vi "imp_test_v3.vi"() -> ()   [LabVIEW 2014]
uses:
  <vilib>/LabVIEW Targets/FPGA/cRIO/shared/nicrio_ModuleControls/nicrio_cRIO-9237_DataRatesRing.ctl
  <vilib>/LabVIEW Targets/FPGA/cRIO/shared/nicrio_ModuleControls/nicrio_cRIO-9237_ExcitationVoltageRing.ctl
  <vilib>/rvi/FXPMathLib/FxpSinAndCos/subVIs/nifxpmath_SinAndCos_SimConfig.ctl
  <vilib>/rvi/Emulation/niFpgaGetClockAttributes.vi
  <vilib>/rvi/Emulation/niFpgaSctlEmulationGetInTimedLoop.vi
  <vilib>/rvi/Emulation/niFpgaEmulationReportErrorSimple.vi
  <vilib>/rvi/Emulation/niFpgaProcessEmulError.vi
  <vilib>/rvi/interface/RandomDataEmulation/nirviRandomDataMultiElementFPGAFIFO.vi
  <instcachedir>/0/nirviRandomDataMultiElementFPGAFIFO_AD0CFC12EF974623A9C2E4184BC062B2.lvgen/nirviRandomDataMultiElementFPGAFIFO_AD0CFC12EF974623A9C2E4184BC062B2_023.vi
  <vilib>/rvi/interface/RandomDataEmulation/niFpgaRandomDataHandleErrors.vi
  <vilib>/rvi/Emulation/niFpgaCriticalErrorInLSC.vi
  <vilib>/rvi/eio/common/nirviEmuTemplateMethod_errors.vi
  <vilib>/rvi/FXPMathLib/FxpSinAndCos/simVIs/DllFxpSinAndCosTemp_sub.vi
  <vilib>/rvi/eio/common/nirviEmuTemplatePropertySet_errors.vi
  <vilib>/rvi/DataTransferAndStorage/Container/XNode/niFpgaContainer.xnode
  <vilib>/rvi/interface/RandomDataEmulation/nirviRandomDataFpgaMultiElementTemplate.vi
  <vilib>/eio/EIONode/EIONode.xnode
  <vilib>/rvi/FXPMathLib/FxpMul/XNode/nifxpmath_Multiplier.xnode
  <vilib>/rvi/FXPMathLib/FxpSinAndCos/XNode/nifxpmath_SinAndCos.xnode
  <vilib>/rvi/Analysis/measure/butterworth/XNode/niFpgaButterworthFilter.xnode
  <vilib>/rvi/FXPMathLib/FxpSub/XNode/nifxpmath_Sub.xnode
  <vilib>/rvi/FXPMathLib/FxpAdd/XNode/nifxpmath_Add.xnode
  <vilib>/eio/EIOPropertyNode/EIOPropertyNode.xnode
  <vilib>/rvi/eio/common/nirviEmuTemplatePropertyGet_errors.vi
  <vilib>/rvi/eio/common/nirviEmuTemplatePropertyGet_noerrors.vi
  <vilib>/rvi/eio/common/nirviEmuTemplatePropertySet_noerrors.vi
  <vilib>/rvi/FXPMathLib/sim/FxpSim.dll
panel:
  out "Strain (mf)":fxp<+/-,36,8>
  in  "Strain mean coeff.":i32[](array[numeric])=[-898916953, 1957103773, 3888751]
  out "Dr_for":fxp<+/-,39,10>
  in  "Command type":i16(ring) items=["Step", "Sine"]
  out "Strain (mean)":fxp<+/-,32,4>
  in  "Strain selection":i16(ring) items=["Raw strain", "Mean strain", "Mean strain (f)", "Filtered strain"]
  in  "ft_d or dt_d2":i16(ring) items=["ft_d", "ft_d2"]
  out "vb":fxp<+/-,38,8>
  out "va":fxp<+/-,38,8>
  out "ft_d2":fxp<+/-,64,59>
  out "Force_r":fxp<+/-,64,42>
  in  "Bv":fxp<+/-,22,8>
  out "D_error_dd":fxp<+/-,64,49>
  out "D_error_d":fxp<+/-,33,10>
  in  "Kv":fxp<+/-,22,8>
  out "D_error":fxp<+/-,64,33>
  out "Dr_sin_dd":fxp<+/-,64,48>
  out "Dr_sin_d":fxp<+/-,64,17>
  out "Sin omega":fxp<+/-,52,9>
  out "Dr_sin":fxp<+/-,39,10>
  in  "Sin offset":fxp<+/-,38,9>
  in  "Sin magnitude":fxp<+/-,22,7>
  out "Time now(s)":fxp<+,52,14>
  in  "Sin wave freq. (Hz)":fxp<+/-,32,6>
  in  "Dr_step":fxp<+/-,22,7>
  in  "Drive mode":i16(ring) items=["Backward", "Forward"]
  in  "ft_d coeff.":i32[](array[numeric])=[946630756, 63555534]
  out "ft_d":fxp<+/-,36,25>
  out "D_dd":fxp<+/-,36,24>
  in  "D_dd coeff.":i32[](array[numeric])=[946630756, 63555534]
  out "dF_PID":fxp<+/-,36,33>
  in  "dF_PID coeff.":i32[](array[numeric])=[946630756, 63555534]
  out "ft_i":fxp<+/-,34,18>
  out "F_PID":fxp<+/-,51,14>
  in  "f_tolorance":fxp<+,22,6>
  in  "Ki":fxp<+/-,36,9>
  in  "Kd":fxp<+/-,36,9>
  out "f_tilde":fxp<+/-,33,11>
  in  "Kp":fxp<+/-,36,9>
  out "vq_F":fxp<+/-,20,5> format="%.57g"
  out "vd_F":fxp<+/-,20,5>
  in  "dF_add":bool
  out "D_d(mm/s)":fxp<+/-,41,10>
  out "omega(rad/s)":fxp<+/-,20,9>
  in  "Veolcity Estimation":i16(ring) items=["T method", "M_avg method", "M method"]
  in  "Stop motor":bool
  out "D_d(T)":fxp<+/-,41,10>
  out "omega(T)":fxp<+/-,20,9>
  in  "mt0_omega":u32
  out "mt_omega":u32
  out "rad(NrTheta)":fxp<+/-,33,20>
  out "D(mm)":fxp<+/-,32,10>
  out "Encoder Position":i32
  in  "Encoder reset":bool
  in  "Ini coe.":bool
  out "Loop rate (kHz)":fxp<+/-,36,7>
  in  "Strain filter coeff.":i32[](array[numeric])=[-850883994, 1909449570, 3794062, -975456236, 2033039520, 4039635]
  out "Force":fxp<+/-,32,10>
  out "Strain (filter)":fxp<+/-,36,4>
  out "Fileterd data":fxp<+/-,32,4>
  in  "S/F coeff":fxp<+/-,20,-12>
  out "Raw Strain":fxp<+/-,36,4>
  in  "Strain gage reset":bool
  in  "Stop (Strain)":bool
  out "Mod6/AI2":fxp<+/-,32,4>
  in  "Shunt Cal Enable":bool
  in  "Half-Bridge Enable":bool
  in  "Excitation Voltage":T1 items=["2.5 Volts", "3.3 Volts", "5.0 Volts", "10.0 Volts", "External Excitation"]
  in  "Data Rate":T2=1 items=["50.000 kS/s (NI 9237)"=1, "25.000 kS/s (NI 9237)"=2, "16.667 kS/s (NI 9237)"=3, "12.500 kS/s (NI 9237)"=4, "10.000 kS/s (NI 9237)"=5, "8.333 kS/s (NI 9237)"=6, "7.143 kS/s (NI 9237)"=7, "6.250 kS/s (NI 9237)"=8, "5.556 kS/s (NI 9237)"=9, "5.000 kS/s (NI 9237)"=10, "4.545 kS/s (NI 9237)"=11, "4.167 kS/s (NI 9237)"=12, "3.846 kS/s (NI 9237)"=13, "3.571 kS/s (NI 9237)"=14, "3.333 kS/s (NI 9237)"=15, "3.125 kS/s (NI 9237)"=16, "2.941 kS/s (NI 9237)"=17, "2.778 kS/s (NI 9237)"=18, "2.632 kS/s (NI 9237)"=19, "2.500 kS/s (NI 9237)"=20, "2.381 kS/s (NI 9237)"=21, "2.273 kS/s (NI 9237)"=22, "2.174 kS/s (NI 9237)"=23, "2.083 kS/s (NI 9237)"=24, "2.000 kS/s (NI 9237)"=25, "1.923 kS/s (NI 9237)"=26, "1.852 kS/s (NI 9237)"=27, "1.786 kS/s (NI 9237)"=28, "1.724 kS/s (NI 9237)"=29, "1.667 kS/s (NI 9237)"=30, "1.613 kS/s (NI 9237)"=31]
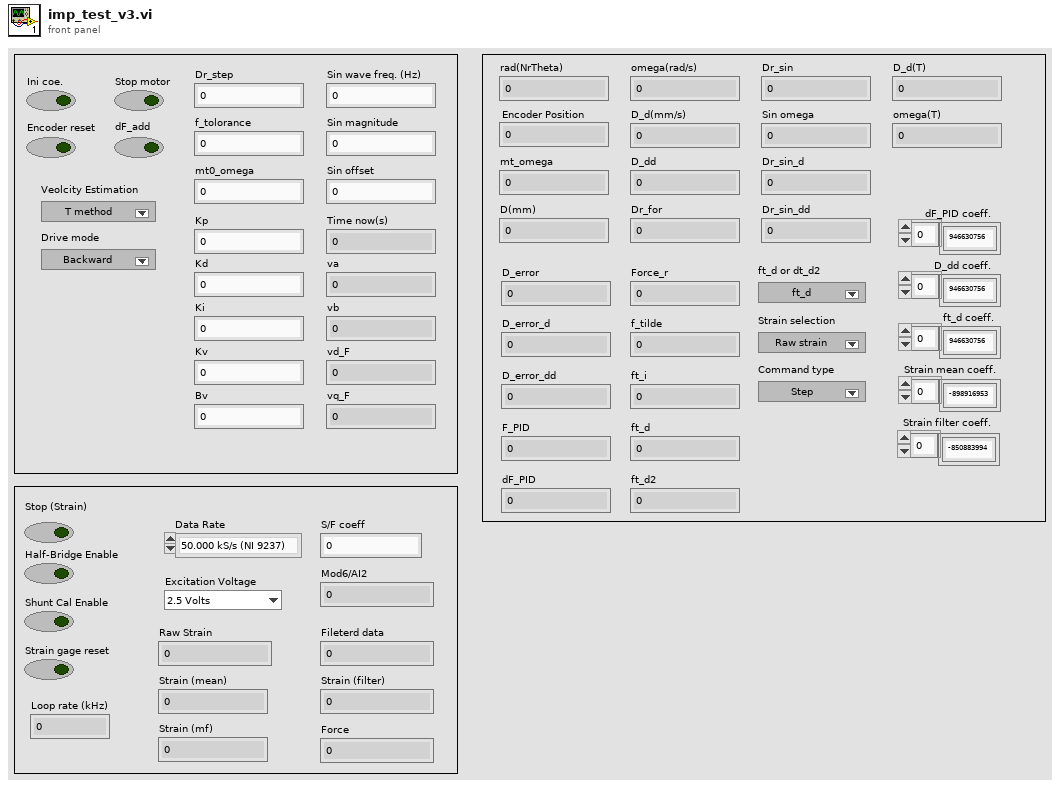
[diagram p1: front panel]
types:
  T1 = typedef "nicrio_cRIO-9237_ExcitationVoltageRing.ctl" = u8
  T2 = typedef "nicrio_cRIO-9237_DataRatesRing.ctl" = u8
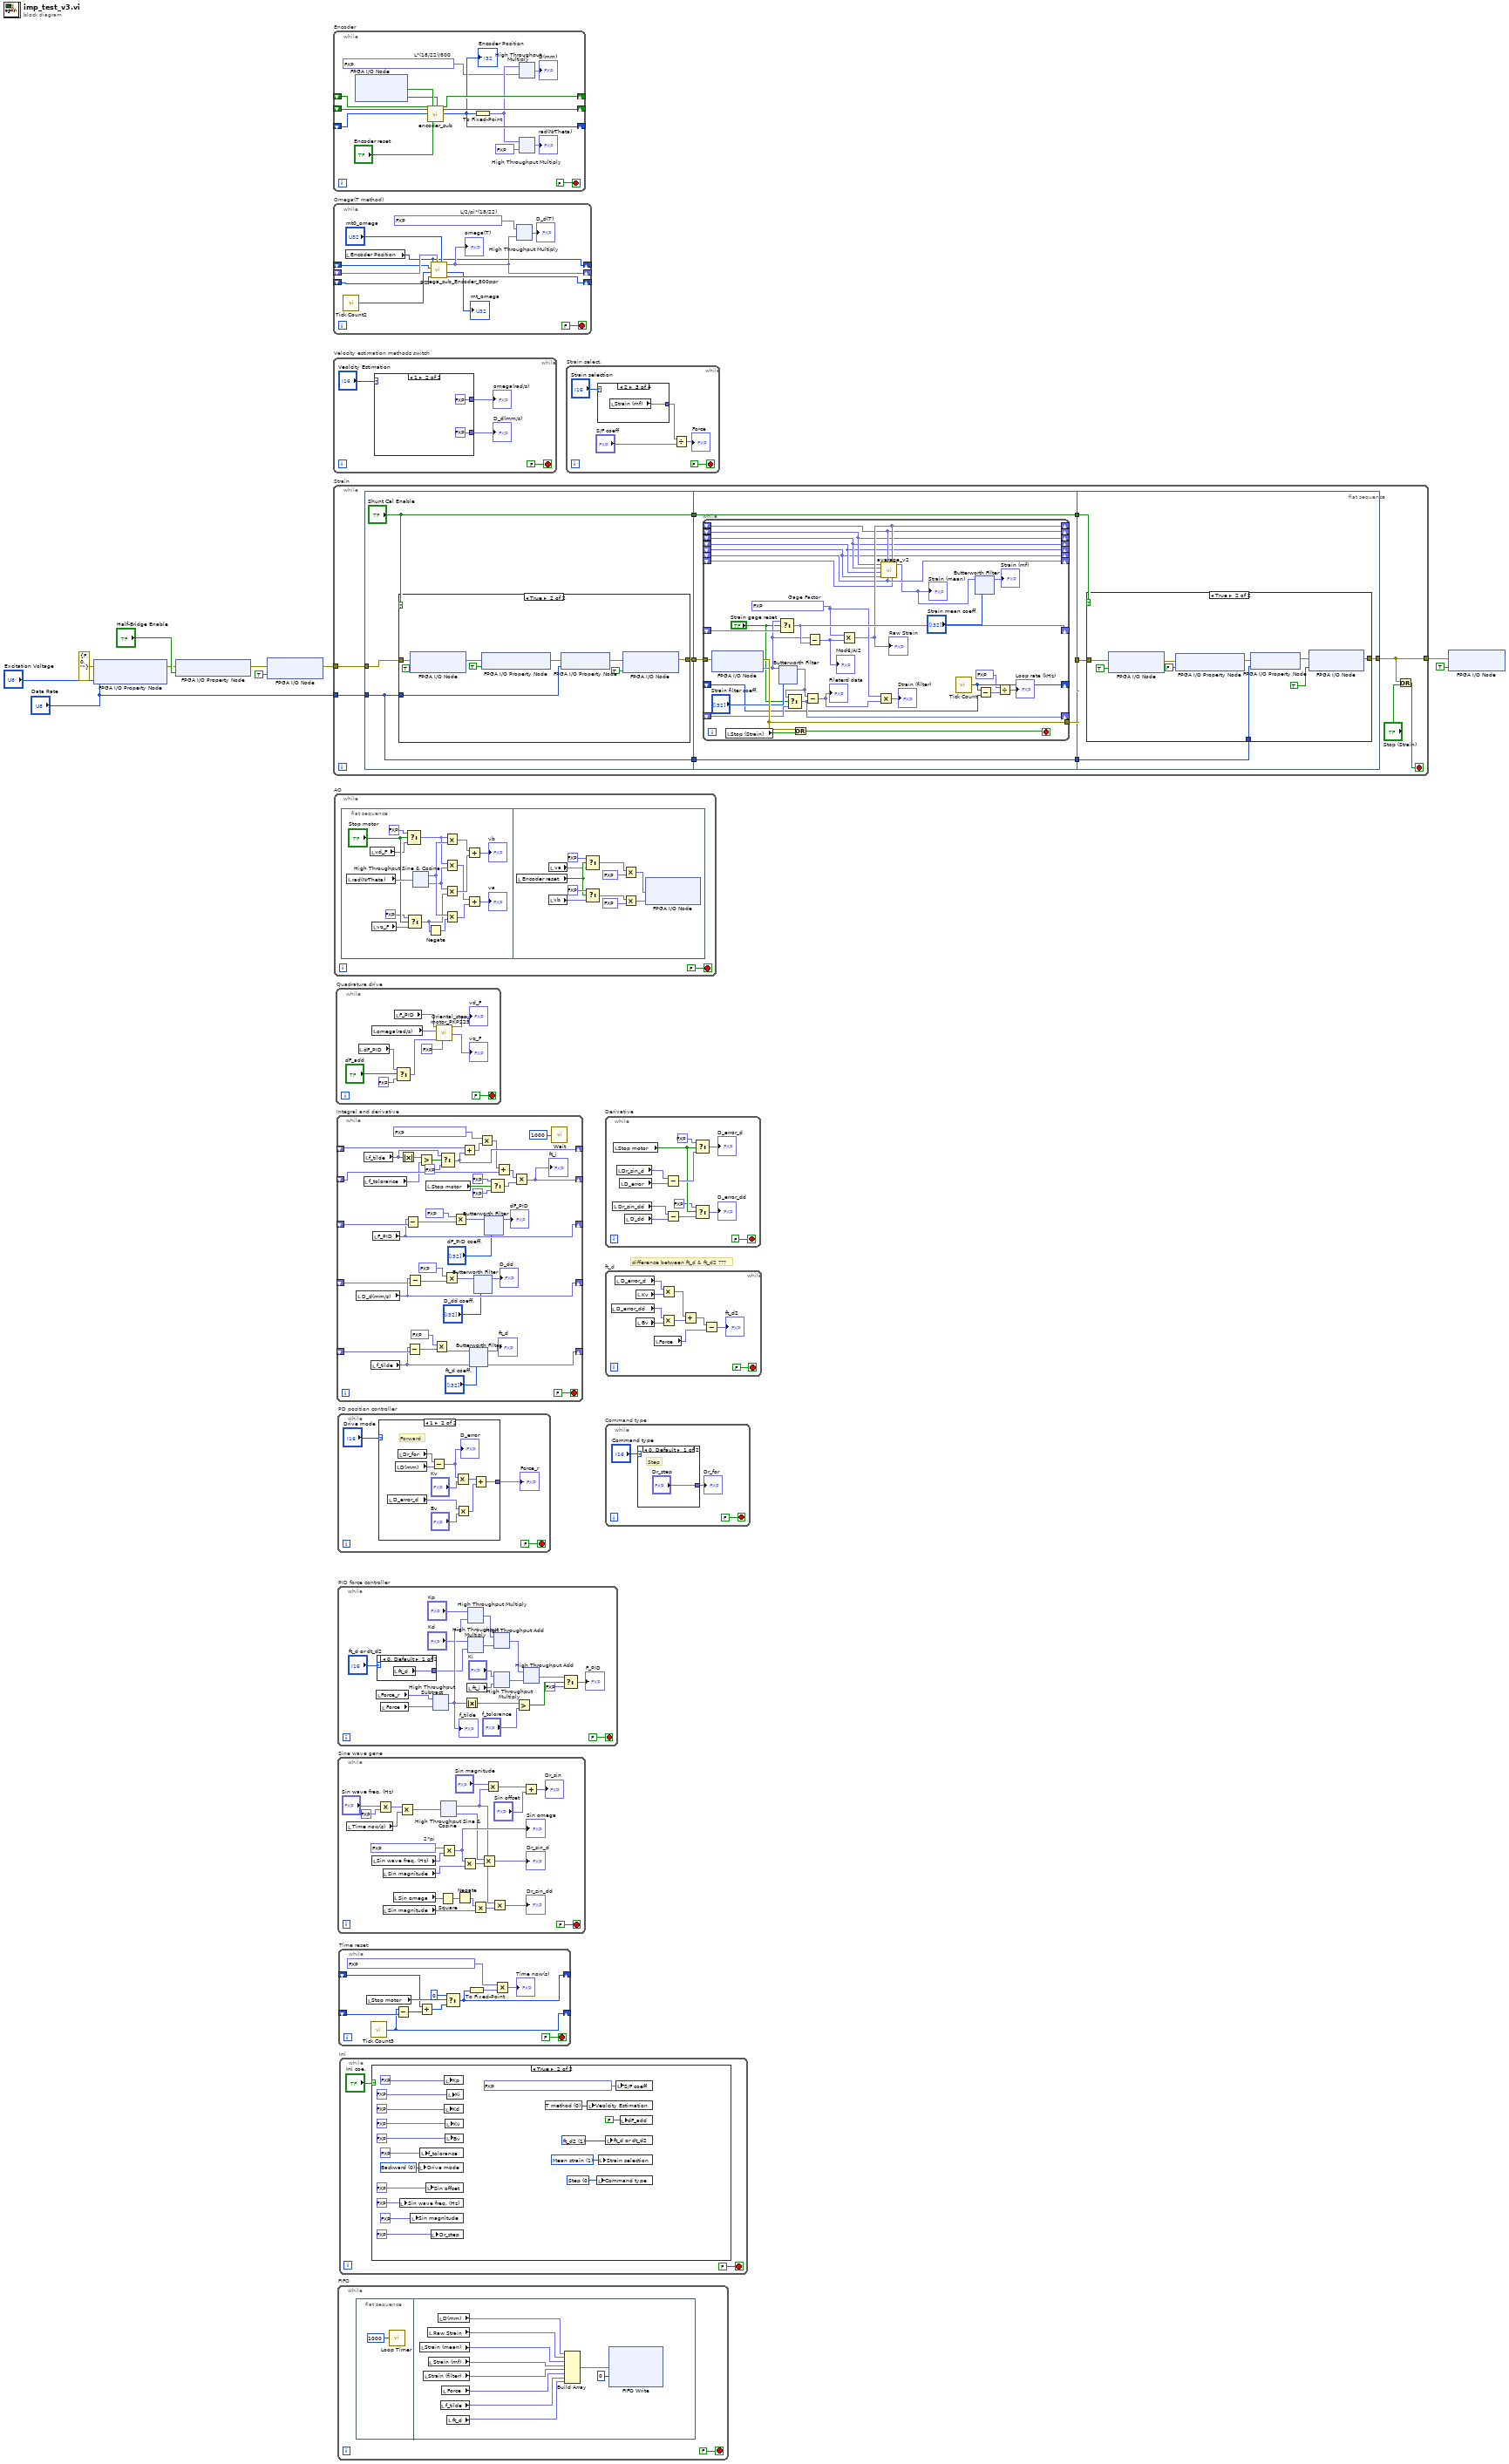
[diagram p0: block diagram]
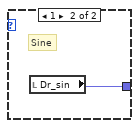
[diagram p2: hidden frame]
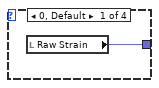
[diagram p3: hidden frame]
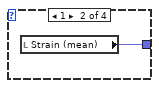
[diagram p4: hidden frame]
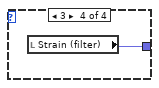
[diagram p5: hidden frame]
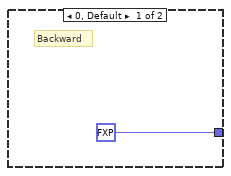
[diagram p6: hidden frame]
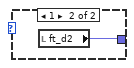
[diagram p7: hidden frame]
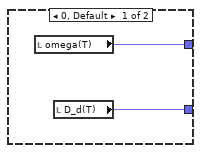
[diagram p8: hidden frame]
diagram:
  # "difference between ft_d & ft_d2 ???"
  n1 = xnode "FPGA I/O Property Node"("error in"=errorcluster {"status"=FALSE, "code"=0, "source"=""}, "Data Rate"="Data Rate", "Excitation Voltage"="Excitation Voltage") -> ("error out"=w7:errorcluster)  [unwired: 1 in, 1 out]
  n2 = xnode "FPGA I/O Property Node"("error in"=w7, "Half-Bridge Enable"="Half-Bridge Enable") -> ("error out"=w6:errorcluster)  [unwired: 1 in, 1 out]
  n3 = xnode "FPGA I/O Node"("error in"=w6, "Mod6/Start"=TRUE) -> ("error out"=w4:errorcluster)  [unwired: 1 in, 1 out]
  n4 = while "Encoder" {
    shift-right: [w22] -> _
    shift-left: _ -> [w23]
    shift-right: [w24] -> _
    shift-left: _ -> [w25]
    shift-right: [w17] -> _
    shift-left: _ -> [w21]
    stop <- FALSE stop-if-true
    w14 = fxp<+/-,32,0> 0.0020454544574022293  # L*(18/22)/800
    n5 = xnode "FPGA I/O Node"() -> ("Mod4/DI3"=w20:bool, "Mod4/DI4"=w19:bool)  [unwired: 2 in, 2 out]
    n6 = call "encoder_sub.vi"("A_pre"=w23, "B_pre"=w25, "Encoder Position_pre"=w21, "A input"=w20, "Encoder Position Reset"="Encoder reset", "B input"=w19) -> ("A"=w22:bool, "B"=w24:bool, "Encoder Position (Counts)"=w17:i32)  [unwired: 19 in]
    "Encoder Position" <- w17
    n7 = To Fixed-Point(number=w17) -> (fixed-point=w16:fxp<+/-,32,32>)  [unwired: 1 in]
    n8 = xnode ("High Throughput Multiply")("x"=w16, "y"=w14) -> ("x*y"=→"D(mm)":fxp<+/-,64,32>)
    n9 = xnode ("High Throughput Multiply")("x"=w16, "y"=fxp<+/-,16,1> 0.125) -> ("x*y"=→"rad(NrTheta)":fxp<+/-,48,33>)
  }
  n10 = while "Omega(T method)" {
    shift-right: [w27] -> _
    shift-left: _ -> [w28]
    shift-right: [w31] -> _
    shift-left: _ -> [w33]
    shift-right: [w35] -> _
    shift-left: _ -> [w36]
    stop <- FALSE stop-if-true
    w30 = fxp<+/-,32,0> 0.2604353614151478  # L/2/pi*(18/22)
    n11 = call "Tick Count2"() -> ("Tick Count(Ticks)"=w37:u32)
    n12 = local read "Encoder Position"() -> (w27:i32)
    n13 = call "omega_sub_Encoder_800ppr.vi"("mt0"="mt0_omega", "omega_pre"=w33, "ticks_m_pre"=w36, "ticks"=w37, "count_pre"=w28, "count"=w27) -> ("ticks_m"=w35:u32, "mt"=→"mt_omega":u32, "omega"=w31:fxp<+/-,20,9>)  [unwired: 3 in]
    "omega(T)" <- w31
    n14 = xnode ("High Throughput Multiply")("x"=w30, "y"=w31) -> ("x*y"=→"D_d(T)":fxp<+/-,52,9>)
  }
  n15 = while "Velocity estimation methods switch" {
    stop <- FALSE stop-if-true
    n16 = case shown="1" "Veolcity Estimation" {
      tunnel: [w43 fxp<+/-,20,9> 0.0 ("omega(T)")] -> w40
      tunnel: [w42 fxp<+/-,41,10> 0.0 ("D_d(T)")] -> w39
      frame 0, Default {
        n17 = local read "omega(T)"() -> (w43:fxp<+/-,20,9>)
        n18 = local read "D_d(T)"() -> (w42:fxp<+/-,41,10>)
      }
      frame 1 {
      }
    }
    "omega(rad/s)" <- w40
    "D_d(mm/s)" <- w39
  }
  n19 = while "Strain" {
    tunnel: w4 -> [w56]
    tunnel: "Data Rate" -> [w55]
    tunnel: [w47] -> w2
    stop <- w48 stop-if-true
    n20 = flat-sequence {
      tunnel: w56 -> [w60]
      tunnel: w55 -> [w59]
      tunnel: [w59] -> w54
      tunnel: ["Shunt Cal Enable"] -> w53
      tunnel: [w57] -> w52
      tunnel: w54 -> [w72]
      tunnel: w53 -> [w73]
      tunnel: w52 -> [w74]
      tunnel: [w73] -> w51
      tunnel: [w71] -> w50
      tunnel: [w72] -> w49
      tunnel: w51 -> [w126]
      tunnel: w50 -> [w125]
      tunnel: w49 -> [w124]
      tunnel: [w123] -> w47
      frame #0 {
        n21 = case shown="True" "Shunt Cal Enable" {
          tunnel: w60 -> [w61 w68]
          tunnel: w59 -> [_ w66]
          tunnel: [w61 w63] -> w57
          frame False {
          }
          frame True {
            n22 = xnode "FPGA I/O Node"("error in"=w68, "Mod6/Stop"=TRUE) -> ("error out"=w69:errorcluster)  [unwired: 1 in, 1 out]
            n23 = xnode "FPGA I/O Property Node"("error in"=w69, "Shunt Cal Enable"=TRUE) -> ("error out"=w67:errorcluster)  [unwired: 1 in, 1 out]
            n24 = xnode "FPGA I/O Property Node"("error in"=w67, "Data Rate"=w66) -> ("error out"=w65:errorcluster)  [unwired: 1 in, 1 out]
            n25 = xnode "FPGA I/O Node"("error in"=w65, "Mod6/Start"=TRUE) -> ("error out"=w63:errorcluster)  [unwired: 1 in, 1 out]
          }
        }
      }
      frame #1 {
        n26 = while {
          tunnel: w74 -> [w106]
          tunnel: [w104] -> w71
          shift-right: [w102] -> _
          shift-left: _ -> [w103]
          shift-right: [w98] -> _
          shift-left: _ -> [w99]
          shift-right: [w90] -> _
          shift-left: _ -> [w91]
          shift-right: [w85] -> _
          shift-left: _ -> [w84]
          shift-right: [w84] -> _
          shift-left: _ -> [w83]
          shift-right: [w83] -> _
          shift-left: _ -> [w82]
          shift-right: [w82] -> _
          shift-left: _ -> [w81]
          shift-right: [w81] -> _
          shift-left: _ -> [w80]
          shift-right: [w80] -> _
          shift-left: _ -> [w79]
          shift-right: [w79] -> _
          shift-left: _ -> [w78]
          stop <- w93 stop-if-true
          w96 = fxp<+,20,2> 2.115001678466797  # Gage Factor
          n27 = xnode "FPGA I/O Node"("error in"=w106) -> ("error out"=w104:errorcluster, "Mod6/AI2"=w100:fxp<+/-,24,-4>)  [unwired: 1 in, 1 out]
          n28 = local read "Stop (Strain)"() -> (w105:bool)
          n29 = xnode "Butterworth Filter"("input data"=w100, "scaled coefficients"="Strain filter coeff.") -> ("output data"=w97:fxp<+/-,28,0>)  [unwired: 1 in]
          n30 = Select(t=w100, s="Strain gage reset", f=w103) -> (s? t:f=w102:fxp<+/-,24,-4>)
          n31 = Select(t=w97, s="Strain gage reset", f=w99) -> (s? t:f=w98:fxp<+/-,28,0>)
          n32 = Or(x=w104, y=w105) -> (x .or. y?=w93:bool)
          n33 = Subtract(x=w97, y=w98) -> (x-y=w95:fxp<+/-,32,16>)
          "Fileterd data" <- w95
          n34 = Subtract(x=w100, y=w102) -> (x-y=w101:fxp<+/-,25,-3>)
          "Mod6/AI2" <- w101
          n35 = Multiply(x=w96, y=w101) -> (x*y=w85:fxp<+/-,41,6>)
          "Raw Strain" <- w85
          n36 = Multiply(x=w96, y=w95) -> (x*y=→"Strain (filter)":fxp<+/-,41,6>)
          n37 = call "average_v2.vi"("Numeric 8"=w78, "Numeric"=w85, "Numeric 7"=w79, "Numeric 2"=w84, "Numeric 6"=w80, "Numeric 5"=w81, "Numeric 4"=w82, "Numeric 3"=w83) -> ("mean"=w77:fxp<+/-,32,4>)  [unwired: 2 in, 1 out]
          "Strain (mean)" <- w77
          n38 = call "Tick Count"() -> ("Tick Count(uSec)"=w90:u32)
          n39 = xnode "Butterworth Filter"("input data"=w77, "scaled coefficients"="Strain mean coeff.") -> ("output data"=→"Strain (mf)":fxp<+/-,32,4>)  [unwired: 1 in]
          n40 = Subtract(x=w90, y=w91) -> (x-y=w88:fxp<+/-,32,16>)
          n41 = Divide(x=fxp<+,7,10> 1000.0, y=w88) -> (x/y=→"Loop rate (kHz)":fxp<+/-,40,27>)
        }
      }
      frame #2 {
        n42 = case shown="True" w126 {
          tunnel: w125 -> [w127 w135]
          tunnel: w124 -> [_ w131]
          tunnel: [w127 w128] -> w123
          frame False {
          }
          frame True {
            n43 = xnode "FPGA I/O Node"("error in"=w135, "Mod6/Stop"=TRUE) -> ("error out"=w133:errorcluster)  [unwired: 1 in, 1 out]
            n44 = xnode "FPGA I/O Property Node"("error in"=w133, "Shunt Cal Enable"=FALSE) -> ("error out"=w132:errorcluster)  [unwired: 1 in, 1 out]
            n45 = xnode "FPGA I/O Property Node"("error in"=w132, "Data Rate"=w131) -> ("error out"=w130:errorcluster)  [unwired: 1 in, 1 out]
            n46 = xnode "FPGA I/O Node"("error in"=w130, "Mod6/Start"=TRUE) -> ("error out"=w128:errorcluster)  [unwired: 1 in, 1 out]
          }
        }
      }
    }
    n47 = Or(x=w47, y="Stop (Strain)") -> (x .or. y?=w48:bool)
  }
  n48 = while "AO" {
    stop <- FALSE stop-if-true
    n49 = flat-sequence {
      frame #0 {
        n50 = local read "rad(NrTheta)"() -> (w154:fxp<+/-,33,20>)
        n51 = local read "vd_F"() -> (w152:fxp<+/-,20,5>)
        n52 = local read "vq_F"() -> (w151:fxp<+/-,20,5>)
        n53 = Select(t=fxp<+/-,20,5> 0.0, s="Stop motor", f=w152) -> (s? t:f=w146:fxp<+/-,20,5>)
        n54 = Select(t=fxp<+/-,20,5> 0.0, s="Stop motor", f=w151) -> (s? t:f=w145:fxp<+/-,20,5>)
        n55 = xnode "High Throughput Sine & Cosine"("x (pi)"=w154) -> ("sin(x)"=w148:fxp<+/-,17,2>, "cos(x)"=w147:fxp<+/-,17,2>)
        n56 = Negate(x=w145) -> (-x=w144:fxp<+/-,21,6>)
        n57 = Multiply(x=w146, y=w148) -> (x*y=w143:fxp<+/-,37,7>)
        n58 = Multiply(x=w146, y=w147) -> (x*y=w141:fxp<+/-,37,7>)
        n59 = Multiply(x=w147, y=w145) -> (x*y=w142:fxp<+/-,37,7>)
        n60 = Multiply(x=w148, y=w144) -> (x*y=w140:fxp<+/-,36,6>)
        n61 = Add(x=w143, y=w142) -> (x+y=→"vb":fxp<+/-,38,8>)
        n62 = Add(x=w141, y=w140) -> (x+y=→"va":fxp<+/-,37,7>)
      }
      frame #1 {
        n63 = local read "Encoder reset"() -> (w187:bool)
        n64 = local read "vb"() -> (w185:fxp<+/-,38,8>)
        n65 = local read "va"() -> (w186:fxp<+/-,38,8>)
        n66 = Select(t=fxp<+,2,2> 3.0, s=w187, f=w186) -> (s? t:f=w191:fxp<+/-,38,8>)
        n67 = Select(t=fxp<+,1,1> 0.0, s=w187, f=w185) -> (s? t:f=w190:fxp<+/-,38,8>)
        n68 = Multiply(x=w191, y=fxp<+/-,1,0> -0.5) -> (x*y=w194:fxp<+/-,39,8>)
        n69 = Multiply(x=w190, y=fxp<+/-,1,0> -0.5) -> (x*y=w195:fxp<+/-,37,6>)
        n70 = xnode "FPGA I/O Node"("Mod8/AO2"=w194, "Mod8/AO3"=w195) -> ()  [unwired: 2 in, 2 out]
      }
    }
  }
  n71 = while "Quadrature drive" {
    stop <- FALSE stop-if-true
    n72 = local read "dF_PID"() -> (w197:fxp<+/-,36,33>)
    n73 = local read "omega(rad/s)"() -> (w205:fxp<+/-,20,9>)
    n74 = local read "F_PID"() -> (w198:fxp<+/-,51,14>)
    n75 = Select(t=w197, s="dF_add", f=fxp<+,1,1> 0.0) -> (s? t:f=w201:fxp<+/-,36,33>)
    n76 = call "Oriental_step_motor_PKP225.vi"("F_Threshold"=fxp<+,12,12> 10.0, "dFmr"=w201, "omega"=w205, "Fmr"=w198) -> ("vq_F"=→"vq_F":fxp<+/-,20,5>, "vd_F"=→"vd_F":fxp<+/-,20,5>)  [unwired: 6 in]
  }
  n77 = while "Integral and derivative" {
    shift-right: [w237] -> _
    shift-left: _ -> [w236]
    shift-right: [w229] -> _
    shift-left: _ -> [w228]
    shift-right: [w239] -> _
    shift-left: _ -> [w240]
    shift-right: [w219] -> _
    shift-left: _ -> [w218]
    shift-right: [w211] -> _
    shift-left: _ -> [w215]
    stop <- FALSE stop-if-true
    n78 = local read "D_d(mm/s)"() -> (w219:fxp<+/-,41,10>)
    n79 = local read "f_tolorance"() -> (w207:fxp<+,22,6>)
    n80 = local read "f_tilde"() -> (w241:fxp<+/-,33,11>)
    n81 = local read "f_tilde"() -> (w211:fxp<+/-,33,11>)
    n82 = local read "F_PID"() -> (w239:fxp<+/-,51,14>)
    n83 = Absolute Value(x=w241) -> (abs(x)=w243:fxp<+,33,11>)
    n84 = Subtract(x=w239, y=w240) -> (x-y=w227:fxp<+/-,52,15>)
    n85 = Subtract(x=w211, y=w215) -> (x-y=w214:fxp<+/-,34,12>)
    n86 = Subtract(x=w219, y=w218) -> (x-y=w221:fxp<+/-,42,11>)
    n87 = Greater?(x=w243, y=w207) -> (0:w244:bool)
    n88 = local read "Stop motor"() -> (w230:bool)
    n89 = Multiply(x=fxp<+/-,33,11> 1000.0, y=w214) -> (x*y=w212:fxp<+/-,64,22>)
    n90 = Select(t=w241, s=w244, f=fxp<+/-,33,11> 0.0) -> (s? t:f=w237:fxp<+/-,33,11>)
    n91 = Multiply(x=fxp<+,7,10> 1000.0, y=w221) -> (x*y=w220:fxp<+/-,49,21>)
    n92 = Multiply(x=fxp<+/-,52,15> 1000.0, y=w227) -> (x*y=w224:fxp<+/-,64,29>)
    n93 = Add(x=w236, y=w237) -> (x+y=w242:fxp<+/-,34,12>)
    n94 = xnode "Butterworth Filter"("input data"=w212, "scaled coefficients"="ft_d coeff.") -> ("output data"=→"ft_d":fxp<+/-,36,26>)  [unwired: 1 in]
    n95 = xnode "Butterworth Filter"("input data"=w220, "scaled coefficients"="D_dd coeff.") -> ("output data"=→"D_dd":fxp<+/-,36,25>)  [unwired: 1 in]
    n96 = Multiply(x=fxp<+/-,30,12> 0.000499725341796875, y=w242) -> (x*y=w235:fxp<+/-,64,24>)
    n97 = xnode "Butterworth Filter"("input data"=w224, "scaled coefficients"="dF_PID coeff.") -> ("output data"=→"dF_PID":fxp<+/-,36,33>)  [unwired: 1 in]
    n98 = Select(t=fxp<+,1,1> 0.0, s=w230, f=fxp<+,1,1> 1.0) -> (s? t:f=w233:fxp<+,1,1>)
    n99 = Add(x=w235, y=w228) -> (x+y=w234:fxp<+/-,64,24>)
    n100 = Multiply(x=w234, y=w233) -> (x*y=w229:fxp<+/-,34,18>)
    "ft_i" <- w229
    n101 = call "Wait"("Count(uSec)"=u32 1000) -> ()  [unwired: 1 out]
  }
  n102 = while "PD position controller" {
    stop <- FALSE stop-if-true
    n103 = case shown="1" "Drive mode" {
      tunnel: [fxp<+/-,62,19> 0.0 w275] -> w271
      frame 0, Default {
        # "Backward"
      }
      frame 1 {
        # "Forward"
        n104 = local read "D_error_d"() -> (w277:fxp<+/-,33,10>)
        n105 = local read "D(mm)"() -> (w282:fxp<+/-,32,10>)
        n106 = local read "Dr_for"() -> (w274:fxp<+/-,39,10>)
        n107 = Subtract(x=w274, y=w282) -> (x-y=w281:fxp<+/-,40,11>)
        "D_error" <- w281
        n108 = Multiply(x=w281, y="Kv") -> (x*y=w279:fxp<+/-,61,18>)
        n109 = Multiply(x=w277, y="Bv") -> (x*y=w276:fxp<+/-,55,18>)
        n110 = Add(x=w279, y=w276) -> (x+y=w275:fxp<+/-,62,19>)
      }
    }
    "Force_r" <- w271
  }
  n111 = while "PID force controller" {
    stop <- FALSE stop-if-true
    n112 = local read "Force_r"() -> (w287:fxp<+/-,64,42>)
    n113 = case shown="0, Default" "ft_d or dt_d2" {
      tunnel: [w303 w304] -> w283
      frame 0, Default {
        n114 = local read "ft_d"() -> (w303:fxp<+/-,36,25>)
      }
      frame 1 {
        n115 = local read "ft_d2"() -> (w304:fxp<+/-,64,59>)
      }
    }
    n116 = local read "Force"() -> (w301:fxp<+/-,32,10>)
    n117 = xnode "High Throughput Subtract"("x"=w287, "y"=w301) -> ("x-y"=w300:fxp<+/-,64,43>)
    "f_tilde" <- w300
    n118 = Absolute Value(x=w300) -> (abs(x)=w291:fxp<+,64,43>)
    n119 = local read "ft_i"() -> (w286:fxp<+/-,34,18>)
    n120 = xnode ("High Throughput Multiply")("x"="Kp", "y"=w300) -> ("x*y"=w298:fxp<+/-,64,52>)
    n121 = xnode ("High Throughput Multiply")("x"="Kd", "y"=w283) -> ("x*y"=w297:fxp<+/-,64,68>)
    n122 = xnode ("High Throughput Add")("x"=w298, "y"=w297) -> ("x+y"=w294:fxp<+/-,64,69>)
    n123 = xnode ("High Throughput Multiply")("x"="Ki", "y"=w286) -> ("x*y"=w295:fxp<+/-,64,27>)
    n124 = Greater?(x=w291, y="f_tolorance") -> (0:w289:bool)
    n125 = xnode ("High Throughput Add")("x"=w294, "y"=w295) -> ("x+y"=w293:fxp<+/-,64,70>)
    n126 = Select(t=w293, s=w289, f=fxp<+/-,51,14> 0.0) -> (s? t:f=→"F_PID":fxp<+/-,64,70>)
  }
  n127 = while "Sine wave gene" {
    stop <- FALSE stop-if-true
    w319 = fxp<+,20,3> 6.2831878662109375  # 2*pi
    n128 = local read "Time now(s)"() -> (w325:fxp<+,52,14>)
    n129 = local read "Sin wave freq. (Hz)"() -> (w318:fxp<+/-,32,6>)
    n130 = Multiply(x="Sin wave freq. (Hz)", y=fxp<+/-,32,6> 2.0) -> (x*y=w326:fxp<+/-,64,12>)
    n131 = local read "Sin magnitude"() -> (w316:fxp<+/-,22,7>)
    n132 = local read "Sin magnitude"() -> (w309:fxp<+/-,22,7>)
    n133 = local read "Sin omega"() -> (w312:fxp<+/-,52,9>)
    n134 = Multiply(x=w326, y=w325) -> (x*y=w324:fxp<+/-,64,25>)
    n135 = Square(x=w312) -> (x^2=w311:fxp<+,64,16>)
    n136 = xnode "High Throughput Sine & Cosine"("x (pi)"=w324) -> ("sin(x)"=w306:fxp<+/-,16,2>, "cos(x)"=w314:fxp<+/-,16,2>)
    n137 = Multiply(x=w319, y=w318) -> (x*y=w317:fxp<+/-,52,9>)
    "Sin omega" <- w317
    n138 = Negate(x=w311) -> (-x=w310:fxp<+/-,64,17>)
    n139 = Multiply(x=w317, y=w316) -> (x*y=w315:fxp<+/-,64,15>)
    n140 = Multiply(x=w310, y=w309) -> (x*y=w308:fxp<+/-,64,24>)
    n141 = Multiply(x=w314, y=w315) -> (x*y=→"Dr_sin_d":fxp<+/-,64,17>)
    n142 = Multiply(x="Sin magnitude", y=w306) -> (x*y=w322:fxp<+/-,38,9>)
    n143 = Multiply(x=w306, y=w308) -> (x*y=→"Dr_sin_dd":fxp<+/-,64,26>)
    n144 = Add(x=w322, y="Sin offset") -> (x+y=→"Dr_sin":fxp<+/-,39,10>)
  }
  n145 = while "FIFO" {
    stop <- FALSE stop-if-true
    n146 = flat-sequence {
      frame #0 {
        n147 = call "Loop Timer"("Count(uSec)"=u32 1000) -> ()  [unwired: 1 out]
      }
      frame #1 {
        n148 = local read "Strain (mean)"() -> (w368:fxp<+/-,32,4>)
        n149 = local read "Strain (filter)"() -> (w366:fxp<+/-,36,4>)
        n150 = local read "Raw Strain"() -> (w369:fxp<+/-,36,4>)
        n151 = local read "Strain (mf)"() -> (w367:fxp<+/-,36,8>)
        n152 = local read "D(mm)"() -> (w370:fxp<+/-,32,10>)
        n153 = local read "f_tilde"() -> (w364:fxp<+/-,33,11>)
        n154 = local read "Force"() -> (w365:fxp<+/-,32,10>)
        n155 = local read "ft_d"() -> (w361:fxp<+/-,36,25>)
        n156 = Build Array(w370, w369, w368, w367, w366, w365, w364, w361) -> (w363:fxp<+/-,57,25>[])
        n157 = xnode ("FIFO Write")("Element"=w363, "Timeout"=0) -> ()  [unwired: 1 in, 2 out]
      }
    }
  }
  n158 = while "Time reset" {
    shift-right: [w380] -> _
    shift-left: _ -> [w381]
    shift-right: [w375] -> _
    shift-left: _ -> [w376]
    stop <- FALSE stop-if-true
    n159 = local read "Stop motor"() -> (w382:bool)
    n160 = call "Tick Count3"() -> ("Tick Count(uSec)"=w380:u32)
    n161 = Subtract(x=w380, y=w381) -> (x-y=w379:u32)
    n162 = Add(x=w376, y=w379) -> (x+y=w378:u32)
    n163 = Select(t=u32 0, s=w382, f=w378) -> (s? t:f=w375:u32)
    n164 = To Fixed-Point(number=w375) -> (fixed-point=w374:fxp<+,32,32>)  [unwired: 1 in]
    n165 = Multiply(x=fxp<+,20,-18> 1.0000003385357559e-06, y=w374) -> (x*y=→"Time now(s)":fxp<+,52,14>)
  }
  n166 = while "Ini" {
    stop <- FALSE stop-if-true
    n167 = case shown="True" "Ini coe." {
      frame False {
      }
      frame True {
        w385 = i16 1 items=["Raw strain", "Mean strain", "Mean strain (f)", "Filtered strain"] ("Strain selection")
        w386 = i16 0 items=["Step", "Sine"] ("Command type")
        w387 = i16 1 items=["ft_d", "ft_d2"] ("ft_d or dt_d2")
        w393 = i16 0 items=["T method", "M_avg method", "M method"] ("Veolcity Estimation")
        w395 = i16 0 items=["Backward", "Forward"] ("Drive mode")
        n168 = local write "Sin wave freq. (Hz)"(fxp<+/-,32,6> 1.0 ("Sin wave freq. (Hz)")) -> ()
        n169 = local write "Sin magnitude"(fxp<+/-,22,7> 10.0 ("Sin magnitude")) -> ()
        n170 = local write "Drive mode"(w395) -> ()
        n171 = local write "f_tolorance"(fxp<+,22,6> 10.0 ("f_tolorance")) -> ()
        n172 = local write "Sin offset"(fxp<+/-,38,9> 0.0 ("Sin offset")) -> ()
        n173 = local write "Dr_step"(fxp<+/-,22,7> 0.0 ("Dr")) -> ()
        n174 = local write "Kp"(fxp<+/-,36,9> 30.0 ("Kp")) -> ()
        n175 = local write "Kd"(fxp<+/-,36,9> 0.0 ("Kd")) -> ()
        n176 = local write "Kv"(fxp<+/-,22,8> 1.0 ("Kv")) -> ()
        n177 = local write "Bv"(fxp<+/-,22,8> 0.0 ("Bv")) -> ()
        n178 = local write "Ki"(fxp<+/-,36,9> 0.0 ("Ki")) -> ()
        n179 = local write "Veolcity Estimation"(w393) -> ()
        n180 = local write "Command type"(w386) -> ()
        n181 = local write "Strain selection"(w385) -> ()
        n182 = local write "ft_d or dt_d2"(w387) -> ()
        n183 = local write "S/F coeff"(fxp<+/-,41,4> 1.047803380060941e-06 ("S/F coeff")) -> ()
        n184 = local write "dF_add"(FALSE ("dF_add")) -> ()
      }
    }
  }
  n185 = while "Strain select." {
    stop <- FALSE stop-if-true
    n186 = case shown="2" "Strain selection" {
      tunnel: [w407 w408 w409 w410] -> w404
      frame 0, Default {
        n187 = local read "Raw Strain"() -> (w407:fxp<+/-,36,4>)
      }
      frame 1 {
        n188 = local read "Strain (mean)"() -> (w408:fxp<+/-,32,4>)
      }
      frame 2 {
        n189 = local read "Strain (mf)"() -> (w409:fxp<+/-,36,8>)
      }
      frame 3 {
        n190 = local read "Strain (filter)"() -> (w410:fxp<+/-,36,4>)
      }
    }
    n191 = Divide(x=w404, y="S/F coeff") -> (x/y=→"Force":fxp<+/-,32,10>)
  }
  n192 = while "Derivative" {
    stop <- FALSE stop-if-true
    n193 = local read "Dr_sin_dd"() -> (w416:fxp<+/-,64,48>)
    n194 = local read "Stop motor"() -> (w414:bool)
    n195 = local read "Dr_sin_d"() -> (w419:fxp<+/-,64,17>)
    n196 = local read "D_error"() -> (w420:fxp<+/-,64,33>)
    n197 = local read "D_dd"() -> (w417:fxp<+/-,36,24>)
    n198 = Subtract(x=w419, y=w420) -> (x-y=w418:fxp<+/-,64,34>)
    n199 = Subtract(x=w416, y=w417) -> (x-y=w415:fxp<+/-,64,49>)
    n200 = Select(t=fxp<+,1,1> 0.0, s=w414, f=w418) -> (s? t:f=→"D_error_d":fxp<+/-,64,34>)
    n201 = Select(t=fxp<+/-,64,49> 0.0, s=w414, f=w415) -> (s? t:f=→"D_error_dd":fxp<+/-,64,49>)
  }
  n202 = while "ft_d" {
    stop <- FALSE stop-if-true
    n203 = local read "D_error_dd"() -> (w429:fxp<+/-,64,49>)
    n204 = local read "D_error_d"() -> (w431:fxp<+/-,33,10>)
    n205 = local read "Kv"() -> (w432:fxp<+/-,22,8>)
    n206 = local read "Bv"() -> (w430:fxp<+/-,22,8>)
    n207 = local read "Force"() -> (w425:fxp<+/-,32,10>)
    n208 = Multiply(x=w431, y=w432) -> (x*y=w427:fxp<+/-,55,18>)
    n209 = Multiply(x=w429, y=w430) -> (x*y=w428:fxp<+/-,64,57>)
    n210 = Add(x=w427, y=w428) -> (x+y=w426:fxp<+/-,64,58>)
    n211 = Subtract(x=w426, y=w425) -> (x-y=→"ft_d2":fxp<+/-,64,59>)
  }
  n212 = while "Command type" {
    stop <- FALSE stop-if-true
    n213 = case shown="0, Default" "Command type" {
      tunnel: ["Dr_step" w437] -> w434
      frame 0, Default {
        # "Step"
      }
      frame 1 {
        # "Sine"
        n214 = local read "Dr_sin"() -> (w437:fxp<+/-,39,10>)
      }
    }
    "Dr_for" <- w434
  }
  n215 = xnode "FPGA I/O Node"("error in"=w2, "Mod6/Stop"=TRUE) -> ()  [unwired: 1 in, 2 out]
